vi "RichToFlatGreeter_res.vi"(5 "OutputClusterType":T1, 11 "InputCluster":T2) -> (3 "OutputCluster":T1)   [LabVIEW 2019, in "Generated_server.lvlib"]
uses:
  Generated_server.lvlib
  Greeter_res.ctl
  Greeter_res_res_oneof/Greeter_res_res_oneof.lvclass
  Greeter_res_Flat.ctl
  Greeter_res_res_oneof/Greeter_res_res_oneof.lvclass/Greeter_res_res_oneof.ctl
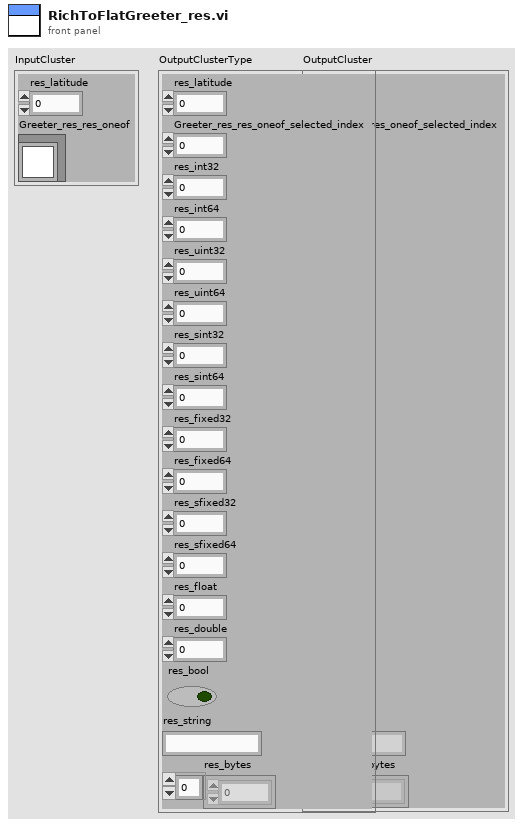
[diagram p1: front panel]
types:
  T1 = typedef "Generated_server.lvlib/Greeter_res_Flat.ctl" = cluster{"res_latitude":i32, "Greeter_res_res_oneof_selected_index":i32, "res_int32":i32, "res_int64":i64, "res_uint32":u32, "res_uint64":u64, "res_sint32":i32, "res_sint64":i64, "res_fixed32":u32, "res_fixed64":u64, "res_sfixed32":i32, "res_sfixed64":i64, "res_float":sgl, "res_double":dbl, "res_bool":bool, "res_string":string, "res_bytes":u8[]}
  T2 = typedef "Generated_server.lvlib/Greeter_res.ctl" = cluster{"res_latitude":i32, "Greeter_res_res_oneof":refnum<class "Greeter_res_res_oneof.lvclass">}
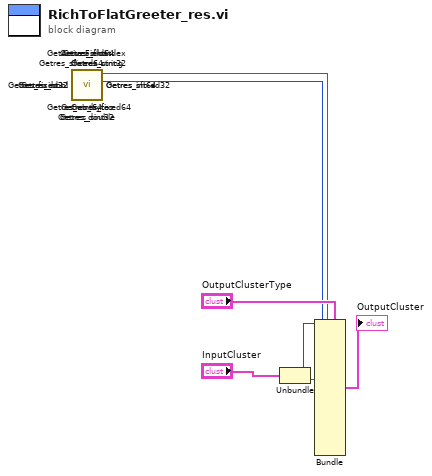
[diagram p0: block diagram]
diagram:
  n1 = Unbundle "Unbundle"("InputCluster") -> ("res_latitude"=w18:i32, "Greeter_res_res_oneof"=w17:refnum<class "Greeter_res_res_oneof.lvclass">)
  n2 = call "Getres_bytes.vi"("OneOfTemplate in"=w17) -> ("Get_Val"=w1:u8[])  [unwired: 8 in, 2 out]
  n3 = call "Getres_string.vi"("OneOfTemplate in"=w17) -> ("Get_Val"=w2:string)  [unwired: 8 in, 2 out]
  n4 = call "Getres_bool.vi"("OneOfTemplate in"=w17) -> ("Get_Val"=w3:bool)  [unwired: 8 in, 2 out]
  n5 = call "Getres_double.vi"("OneOfTemplate in"=w17) -> ("Get_Val"=w4:dbl)  [unwired: 8 in, 2 out]
  n6 = call "Getres_float.vi"("OneOfTemplate in"=w17) -> ("Get_Val"=w5:sgl)  [unwired: 8 in, 2 out]
  n7 = call "Getres_sfixed64.vi"("OneOfTemplate in"=w17) -> ("Get_Val"=w6:i64)  [unwired: 8 in, 2 out]
  n8 = call "Getres_sfixed32.vi"("OneOfTemplate in"=w17) -> ("Get_Val"=w7:i32)  [unwired: 8 in, 2 out]
  n9 = call "Getres_fixed64.vi"("OneOfTemplate in"=w17) -> ("Get_Val"=w8:u64)  [unwired: 8 in, 2 out]
  n10 = call "Getres_fixed32.vi"("OneOfTemplate in"=w17) -> ("Get_Val"=w9:u32)  [unwired: 8 in, 2 out]
  n11 = call "Getres_sint64.vi"("OneOfTemplate in"=w17) -> ("Get_Val"=w10:i64)  [unwired: 8 in, 2 out]
  n12 = call "Getres_sint32.vi"("OneOfTemplate in"=w17) -> ("Get_Val"=w11:i32)  [unwired: 8 in, 2 out]
  n13 = call "Getres_uint64.vi"("OneOfTemplate in"=w17) -> ("Get_Val"=w12:u64)  [unwired: 8 in, 2 out]
  n14 = call "Getres_uint32.vi"("OneOfTemplate in"=w17) -> ("Get_Val"=w13:u32)  [unwired: 8 in, 2 out]
  n15 = call "Getres_int64.vi"("OneOfTemplate in"=w17) -> ("Get_Val"=w14:i64)  [unwired: 8 in, 2 out]
  n16 = call "Getres_int32.vi"("OneOfTemplate in"=w17) -> ("Get_Val"=w15:i32)  [unwired: 8 in, 2 out]
  n17 = call "GetActiveFieldIndex.vi"("OneOfTemplate in"=w17) -> ("Active Field Index"=w16:i32)  [unwired: 8 in, 2 out]
  n18 = Bundle "Bundle"(cluster="OutputClusterType", "res_latitude"=w18, "Greeter_res_res_oneof_selected_index"=w16, "res_int32"=w15, "res_int64"=w14, "res_uint32"=w13, "res_uint64"=w12, "res_sint32"=w11, "res_sint64"=w10, "res_fixed32"=w9, "res_fixed64"=w8, "res_sfixed32"=w7, "res_sfixed64"=w6, "res_float"=w5, "res_double"=w4, "res_bool"=w3, "res_string"=w2, "res_bytes"=w1) -> (→"OutputCluster":T1)
